vi "Resolve Command Linkaging.vi"(7 "Command Refnum in":T2 format="%.0x", 8 "error in (no error)":errorcluster, 10 "Command Format":string, 11 "Linked Channels":T1[](array[typedef]) {"Channel Refnum" format="%.0x"}) -> (0 "error out":errorcluster, 2 "Linked Channels out":T3[](array[typedef]))   [LabVIEW 2018, in "Instrument Addon Scripting API.lvlib"]
uses:
  Instrument Addon Scripting API.lvlib
  Addon/Addon Shared/Types/Linked Channel Cluster.ctl
  <vilib>/NI Veristand/Custom Device API/Custom Device Item Ref.ctl
  TypeDefs/Linked Channel.ctl
  <vilib>/NI VeriStand/Custom Device API/Custom Device API.lvlib
  Addon/Addon Shared/Instrument Addon Shared.lvlib
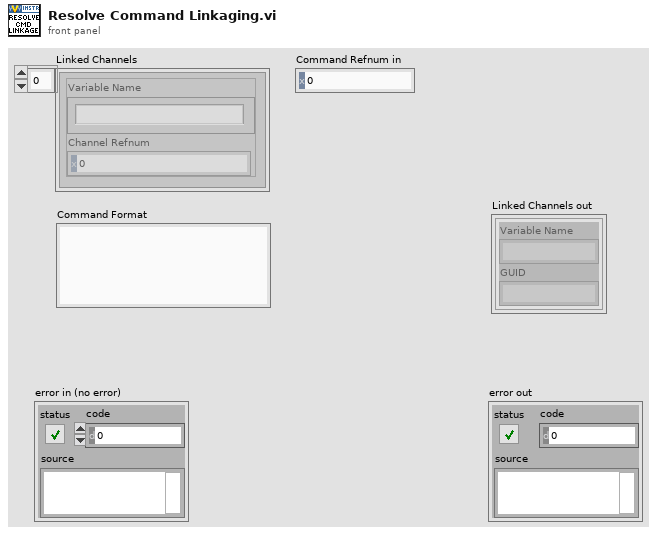
[diagram p1: front panel]
types:
  T1 = typedef "Instrument Addon Scripting API.lvlib/Linked Channel.ctl" = cluster{"Variable Name":string, "Channel Refnum":T2}
  T2 = typedef "Custom Device API.lvlib/Custom Device Item Ref.ctl" = u64
  T3 = typedef "Instrument Addon Shared.lvlib/Linked Channel Cluster.ctl" = cluster{"Variable Name":string, "GUID":string}
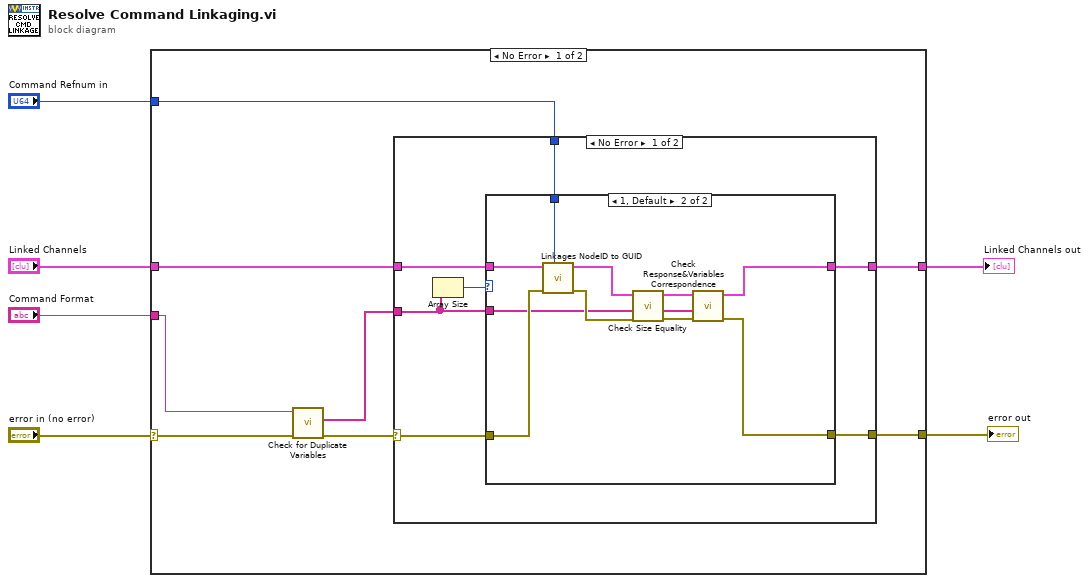
[diagram p0: block diagram]
diagram:
  n1 = case shown="No Error" "error in (no error)" {
    selector: "error in (no error)" -> [w10 w35]
    tunnel: [w14 w35] -> w6
    tunnel: [w13 _] -> w5
    tunnel: "Command Refnum in" -> [w12 _]
    tunnel: "Linked Channels" -> [w11 _]
    tunnel: "Command Format" -> [w9 _]
    frame No Error {
      n2 = call "Check for Duplicate Variables.vi"("error in (no error)"=w10, "Response Format in"=w9) -> ("error out"=w8:errorcluster, "Variables"=w7:string[])  [unwired: 7 in, 1 out]
      n3 = case shown="No Error" w8 {
        selector: w8 -> [w16 w34]
        tunnel: [w21 w34] -> w14
        tunnel: w11 -> [w20 _]
        tunnel: w7 -> [w19 _]
        tunnel: [w18 _] -> w13
        tunnel: w12 -> [w17 _]
        frame No Error {
          n4 = Array Size(array=w19) -> (size(s)=w15:i32)
          n5 = case shown="1, Default" w15 {
            tunnel: w20 -> [_ w33]
            tunnel: w16 -> [w22 w32]
            tunnel: [w22 w29] -> w21
            tunnel: w19 -> [_ w28]
            tunnel: [_ w27] -> w18
            tunnel: w17 -> [_ w26]
            frame 0 {
            }
            frame 1, Default {
              n6 = call "Linkages NodeID to GUID.vi"("Response Refnum in"=w26, "error in (no error)"=w32, "Linked Channels in"=w33) -> ("error out"=w31:errorcluster, "Linked Channels out"=w30:cluster{"Variable Name":string, "GUID":string}[])  [unwired: 7 in]
              n7 = call "Check Size Equality.vi"("Error In"=w31, "Variables"=w28, "Linked Channels in"=w30) -> ("Error Out"=w25:errorcluster, "Variables out"=w23:string[], "Linked Channels out"=w24:cluster{"Variable Name":string, "GUID":string}[])  [unwired: 6 in]
              n8 = call "Check Response&Variables Correspondence.vi"("error in (no error)"=w25, "Variables in"=w23, "Linked Channels in"=w24) -> ("error out"=w29:errorcluster, "Linked Channels out"=w27:T3[])  [unwired: 7 in]
            }
          }
        }
        frame Error {
        }
      }
    }
    frame Error {
    }
  }
  "error out" <- w6
  "Linked Channels out" <- w5
